vi "refnum2string.vi"(11 "Control in":refnum<vi>) -> (3 "String":string)   [LabVIEW 2013]
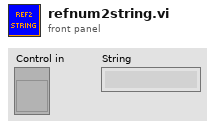
[diagram p1: front panel]
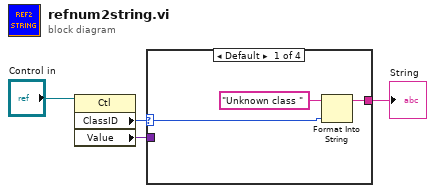
[diagram p0: block diagram]
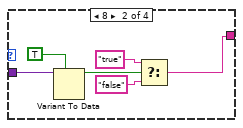
[diagram p2: hidden frame]
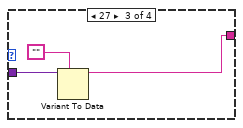
[diagram p3: hidden frame]
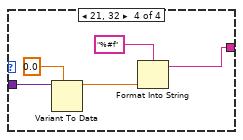
[diagram p4: hidden frame]
diagram:
  n1 = property class="Ctl"(reference="Control in") -> ("ClassID"=w2:u32, "Value"=w4:variant)  [unwired: 1 in, 2 out]
  n2 = case shown="Default" w2 {
    selector: w2 -> [w7 _ _ _]
    tunnel: [w5 w8 w14 w19] -> w3
    tunnel: w4 -> [_ w12 w15 w20]
    frame Default {
      n3 = Format Into String(initial string="Unknown class ", w7) -> (resulting string=w5:string)  [unwired: 2 in, 1 out]
    }
    frame 8 {
      n4 = Variant To Data(type=TRUE, Variant=w12) -> (data=w11:bool)  [unwired: 1 in, 1 out]
      n5 = Select(t="true", s=w11, f="false") -> (s? t:f=w8:string)
    }
    frame 27 {
      n6 = Variant To Data(type="", Variant=w15) -> (data=w14:string)  [unwired: 1 in, 1 out]
    }
    frame 21, 32 {
      n7 = Variant To Data(type=0.0, Variant=w20) -> (data=w18:dbl)  [unwired: 1 in, 1 out]
      n8 = Format Into String(format string="%#f", w18) -> (resulting string=w19:string)  [unwired: 2 in, 1 out]
    }
  }
  "String" <- w3
